vi "Wire Probe.vi"(11 "channel":T1) -> (2 "Value String":string="See Channel Status Window for information.", 3 "Boolean":bool)   [LabVIEW 2020, in "Tag-a[.](c(a[.](stamp),a[.](dbl))).lvlib"]
uses:
  <extravilib>/ChannelInstances/Tag-a[.](c(a[.](stamp),a[.](dbl))).lvlib
  <extravilib>/ChannelInstances/Tag-a[.](c(a[.](stamp),a[.](dbl)))/))Channel.ctl
  <extravilib>/ChannelInstances/Tag-a[.](c(a[.](stamp),a[.](dbl)))/ChannelOp.ctl
  <extravilib>/ChannelInstances/Tag-a[.](c(a[.](stamp),a[.](dbl)))/TagData.lvclass
panel:
  in  "Default Text":string="* If the diagram containing this channel wire has already activated, the channel probe will open immediately.\n\n* Otherwise, the channel probe will open when the diagram that contains this wire probe next activates. To probe a channel from the very beginning of its lifetime, set a wire probe on the channel wire at the highest level diagram where branches from the writers and readers meet up. See \"Probing Channel Wires\" in the LabVIEW help for more information."
  out "Display":string="* If the diagram containing this channel wire has already activated, the channel probe will open immediately.\n\n* Otherwise, the channel probe will open when the diagram that contains this wire probe next activates. To probe a channel from the very beginning of its lifetime, set a wire probe on the channel wire at the highest level diagram where branches from the writers and readers meet up. See \"Probing Channel Wires\" in the LabVIEW help for more information."
  in  "pause on activation?":bool
  in  "Could Not Allocate Probe":string="Could not create probe because of low memory. Please free up memory so that LabVIEW may allocate a channel probe."
  in  "Mismatched Type":string="Could not create probe because of type mismatch. Please alert National Instruments about this error. Until this is repaired, channels of this kind cannot be probed."
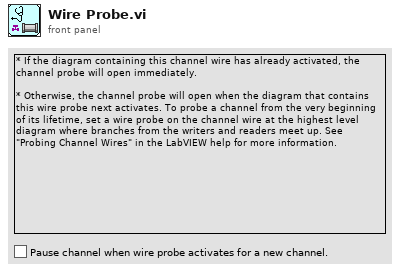
[diagram p1: front panel]
types:
  T1 = typedef "Tag-a[.](c(a[.](stamp),a[.](dbl))).lvlib/))Channel.ctl" = refnum<queue>
  T2 = typedef "Tag-a[.](c(a[.](stamp),a[.](dbl))).lvlib/ChannelOp.ctl" = enum16{"init", "write", "read", "probe"}
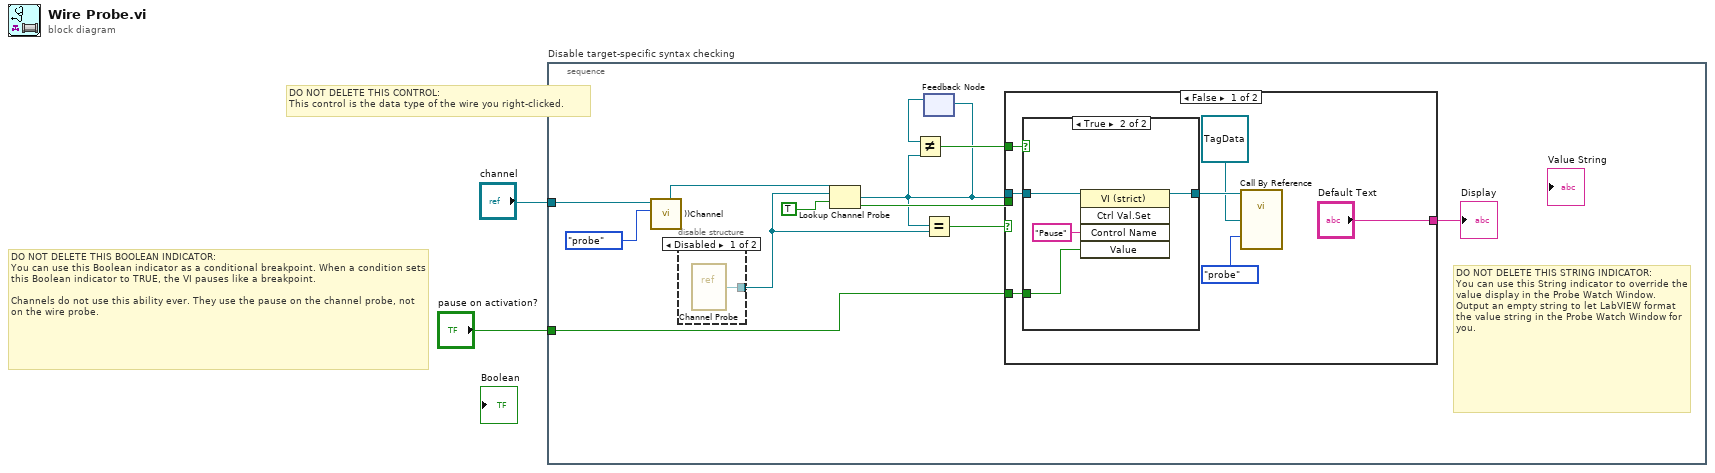
[diagram p0: block diagram]
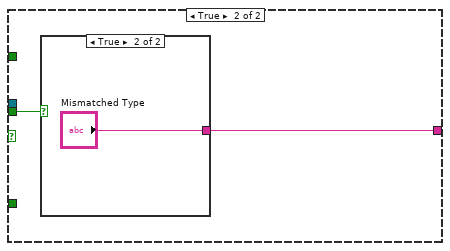
[diagram p4: hidden frame]
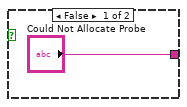
[diagram p5: hidden frame]
diagram:
  # "DO NOT DELETE THIS CONTROL: \nThis control is the data type of the wire you right-clicked."
  # "DO NOT DELETE THIS BOOLEAN INDICATOR: \nYou can use this Boolean indicator as a conditional breakpoint. When a condition sets this Boolean indicator to TRUE, the VI pauses like a breakpoint.\n\nChannels do not use this ability ever. They use the pause on the channel probe, not on the wire probe."
  n1 = stacked-sequence "Disable target-specific syntax checking" {
    tunnel: "channel" -> [w4]
    tunnel: "pause on activation?" -> [w3]
    frame #0 {
      # "DO NOT DELETE THIS STRING INDICATOR: \nYou can use this String indicator to override the value display in the Probe Watch Window.  Output an empty string to let LabVIEW format the value string in the Probe Watch Window for you."
      n2 = call <extravilib>:"))Channel.vi"("channelOp"=ChannelOp."probe", "channel in"=w4) -> ("This VI out"=w6:refnum<vi>)  [unwired: 4 in, 5 out]
      n3 = disable-structure shown="Disabled" {
        disable-tunnel: [w15 _] -> w5
        frame Disabled {
          n4 = vi-ref <extravilib>:"Channel Probe.vi"() -> (w15:refnum<vi>)
        }
        frame Enabled {
        }
      }
      n5 = Lookup Channel Probe(0:w6, 1:w5, 2:TRUE ("force create?")) -> (9:w9:refnum<vi>, 10:w12:bool)
      n6 = feedback #1() -> (w11:refnum<vi>)  [unwired: 1 in]
      n7 = Not Equal?(x=w11, y=w9) -> (x != y?=w10:bool)
      n8 = feedback-in #1(w9) -> ()
      n9 = Equal?(x=w9, y=w5) -> (x = y?=w13:bool)
      n10 = case shown="False" w13 {
        tunnel: w12 -> [_ w29]
        tunnel: ["Default Text" w28] -> w8
        tunnel: w9 -> [w22 _]
        tunnel: w3 -> [w21 _]
        tunnel: w10 -> [w20 _]
        frame False {
          n11 = case shown="True" w20 {
            tunnel: w22 -> [w23 w27]
            tunnel: w21 -> [_ w25]
            tunnel: [w23 w24] -> w19
            frame False {
            }
            frame True {
              n12 = invoke class="VI (strict)" method="Ctrl Val.Set"(reference=w27, "Control Name"="Pause", "Value"=w25) -> (reference out=w24:refnum<vi>)  [unwired: 2 in, 4 out]
            }
          }
          n13 = call-by-ref "?"(reference=w19, "channelOp"=ChannelOp."probe", "tagData in"=refnum<class "TagData.lvclass"> refnum) -> ()  [unwired: 2 in, 3 out]
        }
        frame True {
          n14 = case shown="True" w29 {
            tunnel: ["Could Not Allocate Probe" "Mismatched Type"] -> w28
            frame False {
            }
            frame True {
            }
          }
        }
      }
      "Display" <- w8
    }
  }
